vi "Send Payload.vi"(5 "TCP in":refnum<k5>, 7 "Request Queue":refnum<queue>, 8 "error in (no error)":errorcluster, 9 "SequenceCountService in":refnum<class "SequenceCountService.lvclass">, 10 "source_id":u32, 11 "Send Message Data":T1) -> (0 "error out":errorcluster)   [LabVIEW 2020, in "Vecto.lvlib" / "TCPMessaging.lvclass"]
uses:
  TCPMessaging.lvclass
  Send Message Data.ctl
  proto/TcpPayload/Data.ctl
  SequenceCountService/SequenceCountService.lvclass
  9a68a639-9b61-48b8-9d00-8ce069249e71.vi
  TCPMessaging.lvclass/TCPMessaging.ctl
  proto/TcpPayload/TcpPayload.lvlib
  Vecto.lvlib
  <vilib>/IlluminatedG/IG Promises/Promises/Promise/Promise.lvclass
  Request Registration.ctl
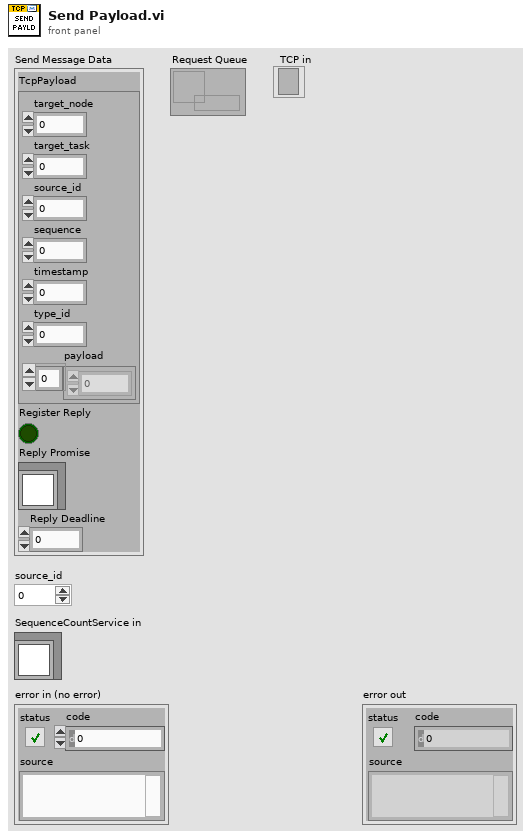
[diagram p1: front panel]
types:
  T1 = typedef "Vecto.lvlib/Send Message Data.ctl" = cluster{"TcpPayload":T2, "Register Reply":bool, "Reply Promise":refnum<class "Promise.lvclass">, "Reply Deadline":dbl}
  T2 = typedef "TcpPayload.lvlib/Data.ctl" = cluster{"target_node":u32, "target_task":u32, "source_id":u32, "sequence":u32, "timestamp":u64, "type_id":u32, "payload":u8[]}
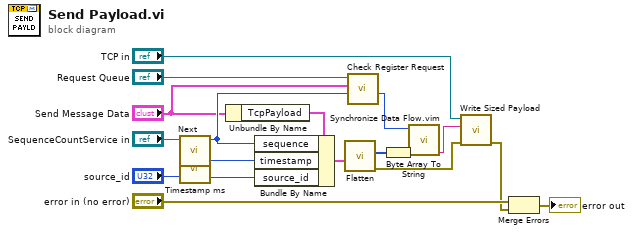
[diagram p0: block diagram]
diagram:
  n1 = call "Next.vi"("SequenceCountService in"="SequenceCountService in") -> ("Sequence"=w5:u32)  [unwired: 9 in, 1 out]
  n2 = call "Timestamp ms.vi"() -> ("Timestamp ms"=w16:u64)  [unwired: 7 in]
  n3 = Unbundle By Name("Send Message Data") -> ("TcpPayload"=w2:T2)
  n4 = Bundle By Name(cluster=w2, "sequence"=w5, "timestamp"=w16, "source_id"="source_id") -> (w3:T2)
  n5 = call "Flatten.vi"("Data"=w3) -> ("error out"=w10:errorcluster, "Buffer"=w17:u8[])  [unwired: 9 in]
  n6 = call "Check Register Request.vi"("Sequence"=w5, "Send Message Data"="Send Message Data", "Request Queue"="Request Queue") -> ("Seq dup"=w1:u32)  [unwired: 8 in]
  n7 = Byte Array To String(unsigned byte array=w17) -> (string=w12:string)
  n8 = call "Synchronize Data Flow.vim"("input 4"=w12, "input 1"=w1) -> ("output 4"=w11:string)  [unwired: 2 in, 3 out]
  n9 = call "Write Sized Payload.vi"("error in (no error)"=w10, "Payload"=w11, "TCP in"="TCP in") -> ("error out"=w8:errorcluster)  [unwired: 7 in, 1 out]
  n10 = Merge Errors("error in (no error)", w8) -> (→"error out":errorcluster)
